vi "send message to server.vi"(8 "error in (no error)":errorcluster, 10 "event message":string, 11 "server in":refnum<class "server.lvclass">) -> (0 "error out":errorcluster, 3 "server out":refnum<class "server.lvclass">)   [LabVIEW 2016, in "server.lvlib" / "server.lvclass"]
uses:
  server.lvclass
  server.lvclass/server.ctl
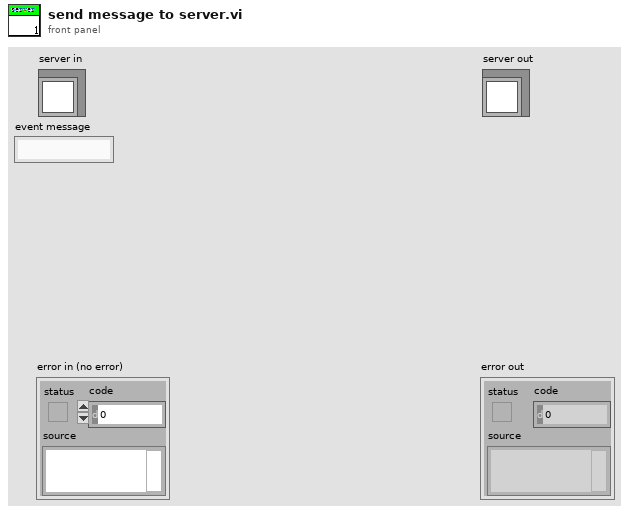
[diagram p1: front panel]
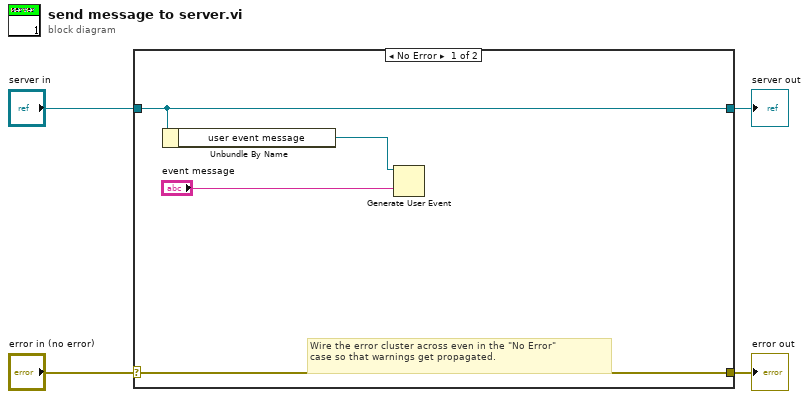
[diagram p0: block diagram]
diagram:
  n1 = case shown="No Error" "error in (no error)" {
    selector: "error in (no error)" -> [w8 w10]
    tunnel: [w8 w10] -> w3
    tunnel: [w7 w9] -> w1
    tunnel: "server in" -> [w7 w9]
    frame No Error {
      # "Wire the error cluster across even in the \"No Error\"\ncase so that warnings get propagated."
      n2 = Unbundle By Name(w7) -> ("user event message"=w6:refnum<user-event>)
      n3 = Generate User Event(user event=w6, event data cluster="event message") -> ()  [unwired: 2 in, 2 out]
    }
    frame Error {
    }
  }
  "error out" <- w3
  "server out" <- w1
